vi "Add Subscriber.vi"(8 "error in (no error)":errorcluster, 10 "New FIFO Instance Config":T1, 11 "CIF_DAQ_DVR_Multi in":refnum<class "CIF_DAQ_DVR_Multi.lvclass">) -> (0 "error out":errorcluster, 2 "New Publisher":string, 3 "CIF_DAQ_DVR_Multi out":refnum<class "CIF_DAQ_DVR_Multi.lvclass">)   [LabVIEW 2021, in "CIF_DAQ_DVR_Multi.lvclass"]
uses:
  CIF_DAQ_DVR_Multi.lvclass
  CIF_DAQ_DVR_Multi.lvclass/CIF_DAQ_DVR_Multi.ctl
  CIFChannels/Typedef/Direction.ctl
  CIFChannels/CIFChannels.lvclass
  ChannelCommon/ChannelCommon.lvlib
  FIFO_DAQ_DVR/CIF_NIChn_FIFO_DAQ_DVR.lvclass
  D:/dev/Packages/Channel_Manager/src/CIF_NIChn/FIFO_DAQ_DVR/CIF_NIChn_FIFO_DAQ_DVR.lvclass
  D:/dev/Packages/Channel_Manager/src/CIF_NIChn/FIFO_U8/CIF_NIChn_Fifo_U8.lvclass
  D:/dev/Packages/Channel_Manager/src/CIF_NIChn/NIChn/CIF_NIChn.lvclass
  D:/dev/Packages/Channel_Manager/src/CIFChannels/CIFChannels.lvclass
  D:/dev/Packages/Channel_Manager/src/CIF_NIChn/FIFO_DAQ_DVR_Multi/CIF_DAQ_DVR_Multi.lvclass
  ChannelCommon/typedef/New FIFO Instance Configuration.ctl
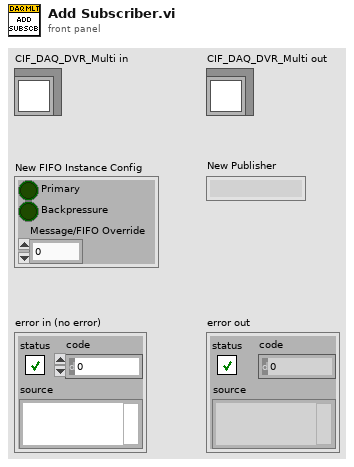
[diagram p1: front panel]
types:
  T1 = typedef "ChannelCommon.lvlib/New FIFO Instance Configuration.ctl" = cluster{"Primary":bool, "Backpressure":bool, "Message/FIFO Override":u32}
  T2 = typedef "CIFChannels.lvclass/Direction.ctl" = enum16{"Publisher", "Subscriber"}
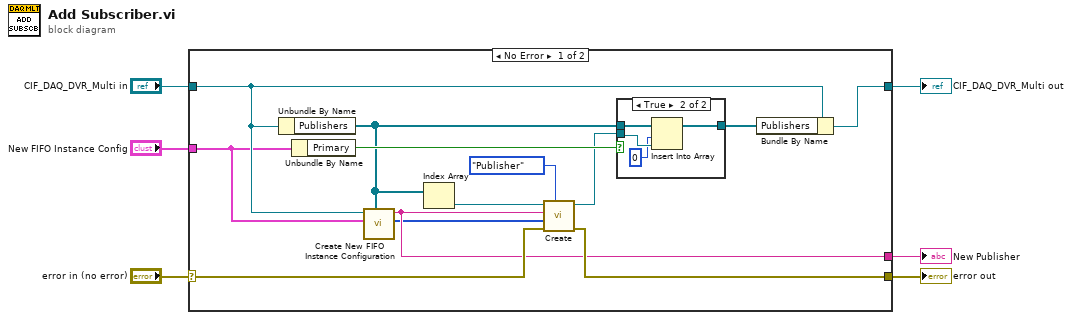
[diagram p0: block diagram]
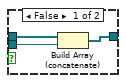
[diagram p2: hidden frame]
diagram:
  n1 = case shown="No Error" "error in (no error)" {
    selector: "error in (no error)" -> [w10 w28]
    tunnel: [w13 w28] -> w5
    tunnel: [w15 w27] -> w3
    tunnel: "CIF_DAQ_DVR_Multi in" -> [w12 w27]
    tunnel: "New FIFO Instance Config" -> [w11 _]
    tunnel: [w9 _] -> w1
    frame No Error {
      n2 = Unbundle By Name(w12) -> ("Publishers"=w7:refnum<class "CIF_NIChn_FIFO_DAQ_DVR.lvclass">[])
      n3 = Unbundle By Name(w11) -> ("Primary"=w17:bool)
      n4 = call "Create New FIFO Instance Configuration.vi"("Publisher Array in"=w7, "New FIFO Instance Config"=w11, "CIFChannels.lvclass"=w12) -> ("Flattened FIFO Config"=w8:u8[], "New Publisher"=w9:string)  [unwired: 7 in]
      n5 = Index Array(array=w7) -> (element=w19:refnum<class "CIF_NIChn_FIFO_DAQ_DVR.lvclass">)  [unwired: 1 in]
      n6 = call-dynamic "Create.vi"("Direction"=Direction."Publisher", "error in (no error)"=w10, "Custom Config Data"=w8, "Name"=w9, "CIF_NIChn_FIFO_DAQ in"=w19) -> ("error out"=w13:errorcluster, "CIF_NIChn_FIFO_DAQ out"=w14:refnum<class "CIF_NIChn_FIFO_DAQ_DVR.lvclass">)  [unwired: 5 in]
      n7 = case shown="True" w17 {
        tunnel: w7 -> [w22 w26]
        tunnel: [w21 w23] -> w16
        tunnel: w14 -> [w20 w25]
        frame False {
          n8 = Build Array (concatenate)(w22, w20) -> (w21:refnum<class "CIF_NIChn_FIFO_DAQ_DVR.lvclass">[])
        }
        frame True {
          n9 = Insert Into Array(array=w26, index=0, new element=w25) -> (w23:refnum<class "CIF_NIChn_FIFO_DAQ_DVR.lvclass">[])
        }
      }
      n10 = Bundle By Name(cluster=w12, "Publishers"=w16) -> (w15:refnum<class "CIF_DAQ_DVR_Multi.lvclass">)
    }
    frame Error {
    }
  }
  "error out" <- w5
  "CIF_DAQ_DVR_Multi out" <- w3
  "New Publisher" <- w1
